vi "Get NIPKG Attributes from VIPM Package File.vi"(6 "Category":string(combo)="Add-Ons", 8 "error in (no error)":errorcluster, 9 "LabVIEW version":string="18.0", 11 "Source VIPM package (.vip)":path) -> (0 "error out":errorcluster, 1 "LabVIEW version out":string="18.0", 2 "package attributes":T1={"Package Name"="", "Display name"="", "Version"="", "Display version"="", "Synopsis"="", "Description"="", "Maintainer"="", "Maintainer email address"="", "Category"="", "Homepage"="", "Release notes"="", "Depends"=[], "Recommends"=[], "Suggests"=[], "Conflicts"=[], "Provides"=[], "Replaces"=[], "Supplements"=[], "Enhances"=[], "Product"=FALSE, "User visible"=FALSE, "Installed size (KB)"=0, "Package filesize (bytes)"=0, "Architecture"="", "Agent"="file", "MD5Checksum"=""}, 3 "VIPM Package Installed Filepaths":path[](array[path]), 4 "VIPM dependencies":string[](array[string]))   [LabVIEW 2014, in "vipm-to-nipm-package-converter.lvlib"]
doc: "From the specified VIPM package (.vip), convert the package attributes into the NIPM package attribute format and return the corresponding NIPM package attributes and return the installed filepaths of the VIPM package.\n\nINPUT(S):\n<b>LabVIEW version</b>: Specifies the LabVIEW version for the NIPM package to support (\"14.0\", \"14.0 (64-bit)\", \"18.0\", \"18.0 (64-bit)\", etc)"
uses:
  vipm-to-nipm-package-converter.lvlib
  <vilib>/National Instruments/NIPM API (Beta)/_support/package attributes.ctl
  <vilib>/Utility/config.llb/Read Key (String).vi
  <vilib>/Utility/config.llb/NI_LVConfig.lvlib
  <vilib>/National Instruments/NIPM API (Beta)/NIPM_API.lvlib
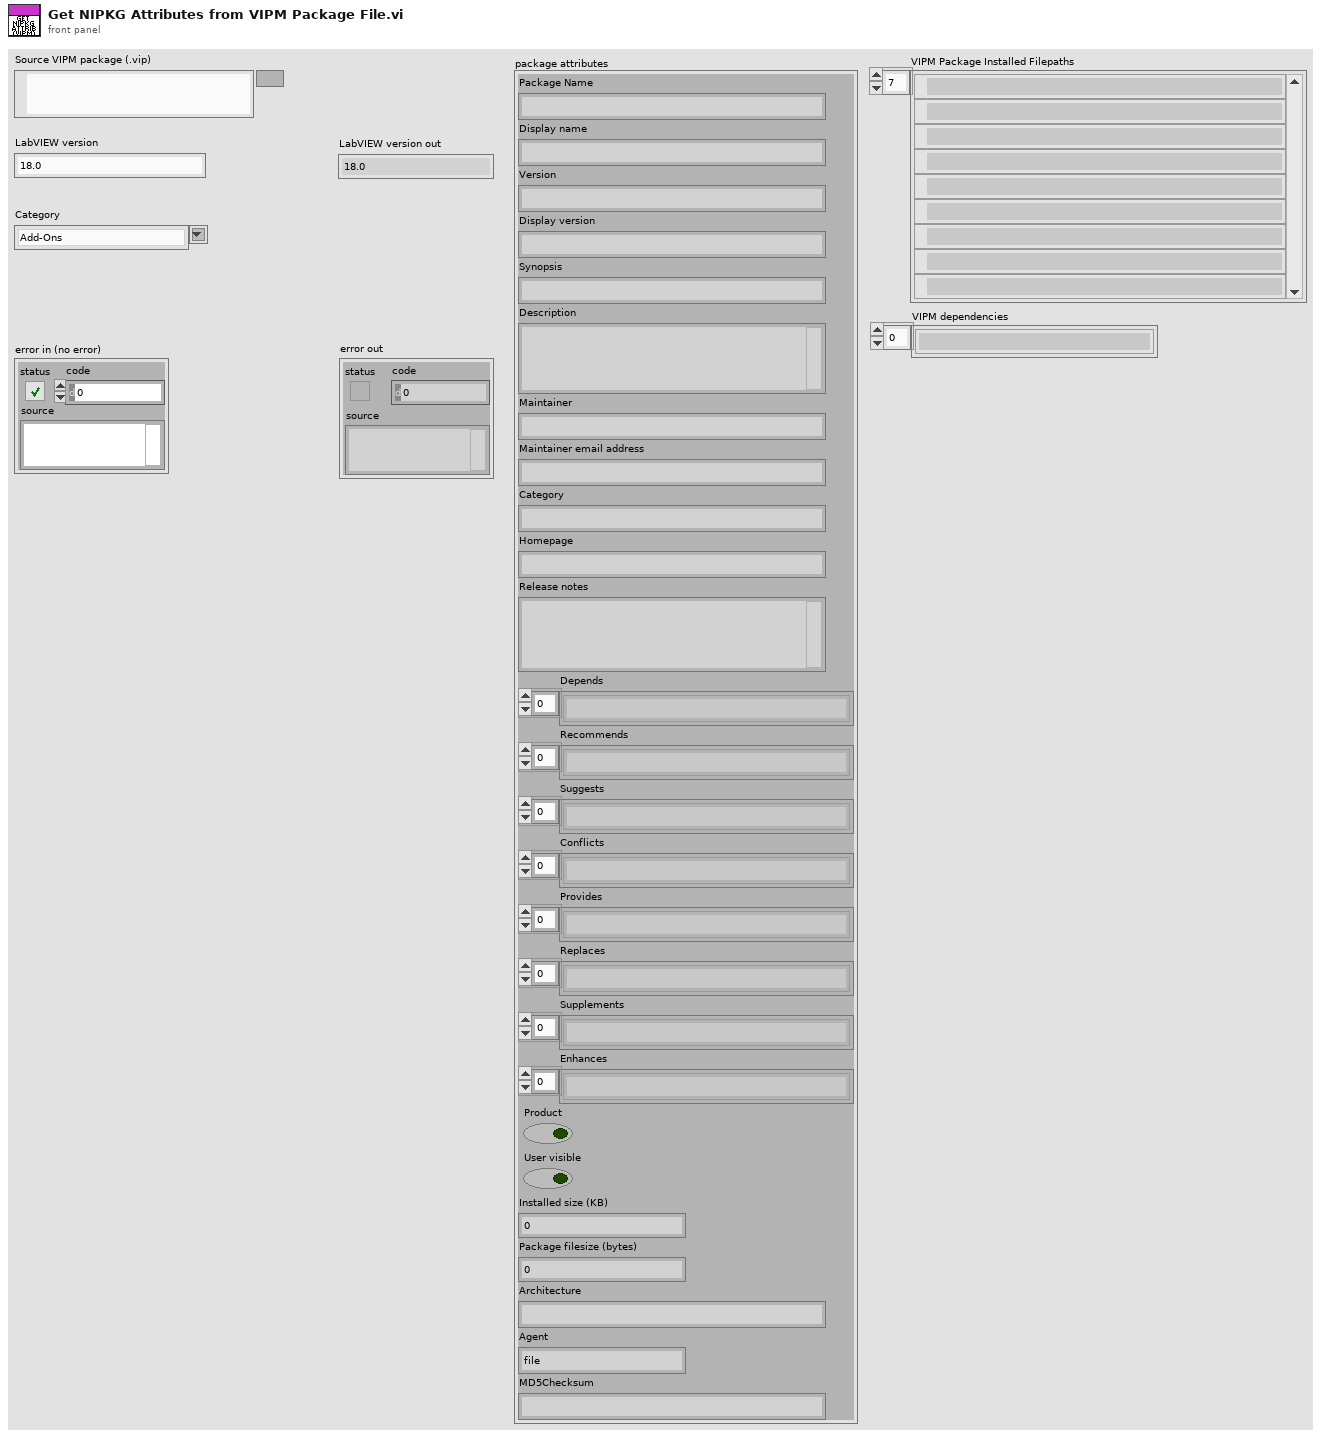
[diagram p1: front panel]
types:
  T1 = typedef "NIPM_API.lvlib/package attributes.ctl" = cluster{"Package Name":string, "Display name":string, "Version":string, "Display version":string, "Synopsis":string, "Description":string, "Maintainer":string, "Maintainer email address":string, "Category":string, "Homepage":string, "Release notes":string, "Depends":string[], "Recommends":string[], "Suggests":string[], "Conflicts":string[], "Provides":string[], "Replaces":string[], "Supplements":string[], "Enhances":string[], "Product":bool, "User visible":bool, "Installed size (KB)":u64, "Package filesize (bytes)":u64, "Architecture":string, "Agent":string, "MD5Checksum":string}
  T2 = typedef "NI_LVConfig.lvlib/Config Data RefNum.ctl" = refnum<k1>
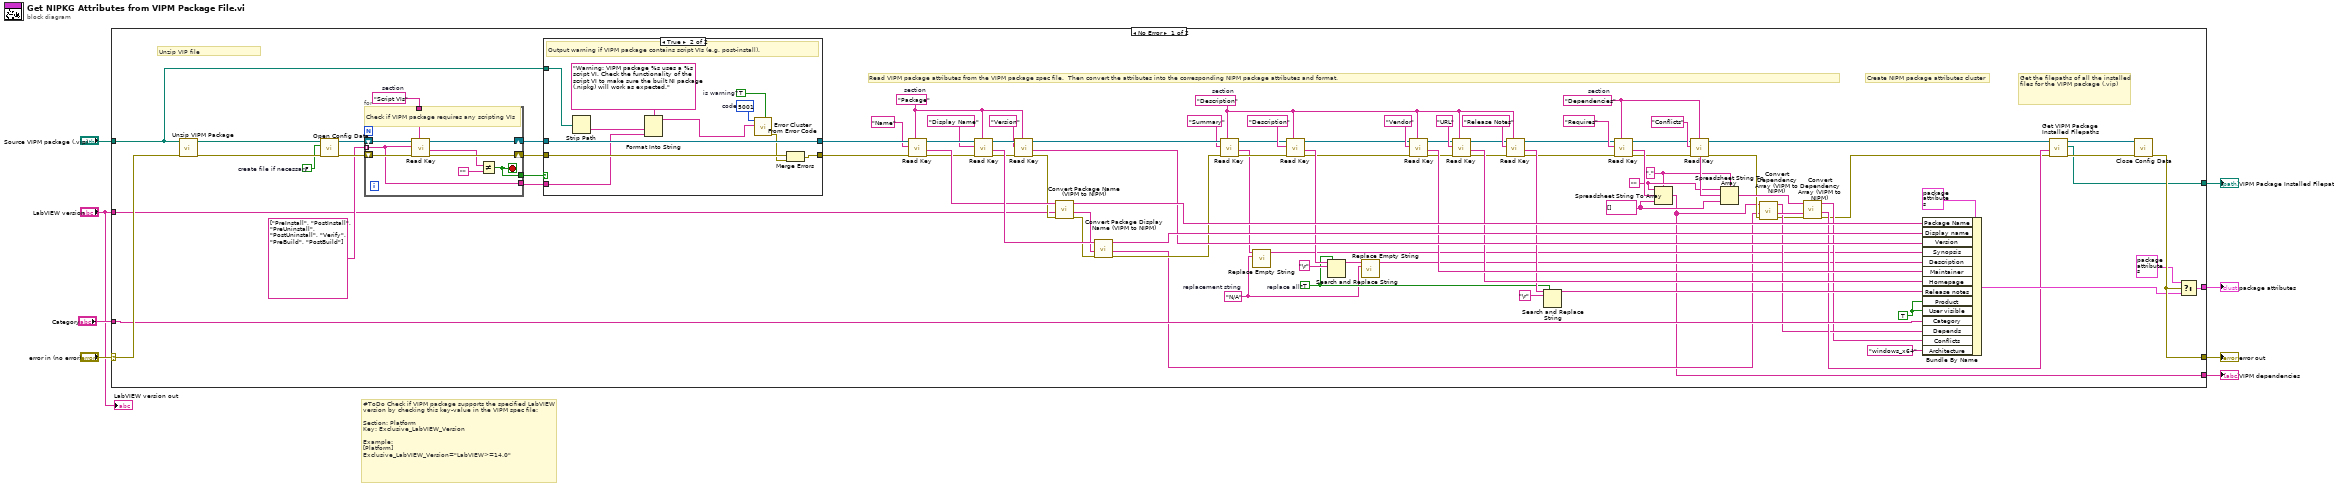
[diagram p0: block diagram]
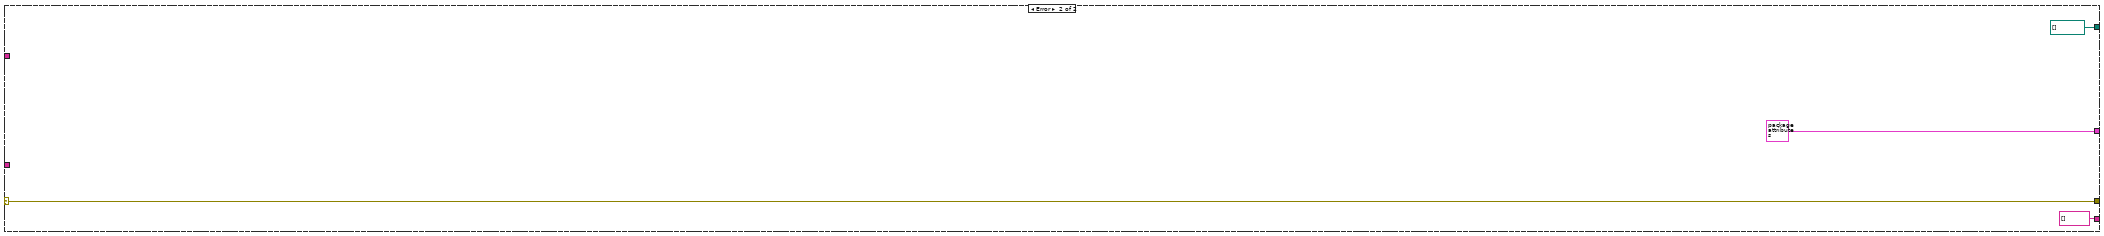
[diagram p3: hidden frame]
diagram:
  # "#ToDo Check if VIPM package supports the specified LabVIEW version by checking this key-value in the VIPM spec file:\n\nSection: Platform\nKey: Exclusive_LabVIEW_Version\n\nExample:\n[Platform]\nExclusive_LabVIEW_Version=\"LabVIEW>=14.0\""
  n1 = case shown="No Error" "error in (no error)" {
    selector: "error in (no error)" -> [w100 w129]
    tunnel: [w93 T1 {"Package Name"="", "Display name"="", "Version"="", "Display version"="", "Synopsis"="", "Description"="", "Maintainer"="", "Maintainer email address"="", "Category"="", "Homepage"="", "Release notes"="", "Depends"=[], "Recommends"=[], "Suggests"=[], "Conflicts"=[], "Provides"=[], "Replaces"=[], "Supplements"=[], "Enhances"=[], "Product"=FALSE, "User visible"=FALSE, "Installed size (KB)"=0, "Package filesize (bytes)"=0, "Architecture"="", "Agent"="file", "MD5Checksum"=""} ("package attributes")] -> w8
    tunnel: "LabVIEW version" -> [w12 _]
    tunnel: "Source VIPM package (.vip)" -> [w81 _]
    tunnel: [w96 w129] -> w6
    tunnel: "Category" -> [w99 _]
    tunnel: [w88 path[] [] ("Installed Filepaths")] -> w2
    tunnel: [w9 string[] []] -> w1
    frame No Error {
      w15 = "N/A"  # replacement string
      w34 = string[] []
      w35 = ""
      w28 = "," ("delimiter (Tab)")
      w39 = "Dependencies"  # section
      w43 = TRUE  # replace all?
      w52 = TRUE ("Product")
      w61 = "Description"  # section
      w72 = "Package"  # section
      w90 = "Script VIs"  # section
      w101 = FALSE  # create file if necessary
      # "Get the filepaths of all the installed files for the VIPM package (.vip)"
      # "Create NIPM package attributes cluster"
      # "Read VIPM package attributes from the VIPM package spec file.  Then convert the attributes into the corresponding NIPM package attributes and format."
      # "Unzip VIP file"
      n2 = call "Unzip VIPM Package.vi"("error in (no error)"=w100, "Source VIPM package (.vip)"=w81) -> ("error out"=w103:errorcluster, "VIPM package spec filepath"=w102:path)  [unwired: 8 in]
      n3 = call <vilib>:"Open Config Data.vi"("error in (no error)"=w103, "create file if necessary (T)"=w101, "configuration file path"=w102) -> ("error out"=w91:errorcluster, "refnum"=w92:T2)  [unwired: 6 in, 1 out]
      n4 = for {
        tunnel: w90 -> [w121]
        shift-right: [w123] -> w86
        shift-left: w92 -> [w125]
        shift-right: [w122] -> w84
        shift-left: w91 -> [w124]
        tunnel: string[] ["PreInstall", "PostInstall", "PreUninstall", "PostUninstall", "Verify", "PreBuild", "PostBuild"] -> [w118] mode=indexing
        tunnel: [w119] -> w87
        tunnel: [w118] -> w82
        stop <- w119 stop-if-true
        # "Check if VIPM package requires any scripting VIs"
        n5 = call-poly <vilib>:"Read Key.vi"("section"=w121, "error in (no error)"=w124, "key"=w118, "refnum"=w125) -> ("error out"=w122:errorcluster, "value"=w117:string, "refnum out"=w123:T2)  [unwired: 4 in, 1 out]
        n6 = Not Equal?(x=w117, y="") -> (x != y?=w119:bool)
      }
      n7 = case shown="True" w87 {
        tunnel: w86 -> [w105 w116]
        tunnel: [w105 w116] -> w85
        tunnel: w84 -> [w104 w115]
        tunnel: [w104 w108] -> w83
        tunnel: w82 -> [_ w111]
        tunnel: w81 -> [_ w112]
        frame False {
          # "VIPM package does not contain any script VIs"
        }
        frame True {
          w106 = TRUE  # is warning?
          w110 = 5001  # code
          # "Output warning if VIPM package contains script VIs (e.g. post-install)."
          n8 = Strip Path(path=w112) -> (name=w114:string)  [unwired: 1 out]
          n9 = Format Into String(format string="Warning: VIPM package %s uses a %s script VI. Check the functionality of the script VI to make sure the built NI package (.nipkg) will work as expected.", w114, w111) -> (resulting string=w109:string)  [unwired: 2 in, 1 out]
          n10 = call <vilib>:"Error Cluster From Error Code.vi"("is warning? (False)"=w106, "error message (\"\")"=w109, "error code (0)"=w110) -> ("error out"=w107:errorcluster)  [unwired: 6 in]
          n11 = Merge Errors(w115, w107) -> (w108:errorcluster)
        }
      }
      n12 = call-poly <vilib>:"Read Key.vi"("section"=w72, "error in (no error)"=w83, "key"="Name", "refnum"=w85) -> ("error out"=w42:errorcluster, "value"=w49:string, "refnum out"=w78:T2)  [unwired: 4 in, 1 out]
      n13 = call-poly <vilib>:"Read Key.vi"("section"=w72, "error in (no error)"=w42, "key"="Display Name", "refnum"=w78) -> ("error out"=w59:errorcluster, "value"=w75:string, "refnum out"=w73:T2)  [unwired: 4 in, 1 out]
      n14 = call-poly <vilib>:"Read Key.vi"("section"=w72, "error in (no error)"=w59, "key"="Version", "refnum"=w73) -> ("error out"=w41:errorcluster, "value"=w70:string, "refnum out"=w69:T2)  [unwired: 4 in, 1 out]
      n15 = call "Convert Package Name (VIPM to NIPM).vi"("error in (no error)"=w41, "LabVIEW version in"=w12, "VIPM Package Name"=w49) -> ("error out"=w51:errorcluster, "LabVIEW version out"=w11:string, "NIPM Package Name"=w76:string)  [unwired: 6 in]
      n16 = call "Convert Package Display Name (VIPM to NIPM).vi"("error in (no error)"=w51, "LabVIEW version in"=w11, "VIPM Package Display Name"=w75) -> ("error out"=w50:errorcluster, "LabVIEW version out"=w10:string, "NIPM Package Display Name"=w74:string)  [unwired: 6 in]
      n17 = call-poly <vilib>:"Read Key.vi"("section"=w61, "error in (no error)"=w50, "key"="Summary", "refnum"=w69) -> ("error out"=w58:errorcluster, "value"=w17:string, "refnum out"=w66:T2)  [unwired: 4 in, 1 out]
      n18 = call "Replace Empty String.vi"("replacement string"=w15, "string in"=w17) -> ("string out"=w16:string)  [unwired: 9 in]
      n19 = call-poly <vilib>:"Read Key.vi"("section"=w61, "error in (no error)"=w58, "key"="Description", "refnum"=w66) -> ("error out"=w18:errorcluster, "value"=w48:string, "refnum out"=w55:T2)  [unwired: 4 in, 1 out]
      n20 = Search and Replace String(replace all?=w43, input string=w48, search string="\r") -> (result string=w14:string)  [unwired: 5 in, 3 out]
      n21 = call "Replace Empty String.vi"("replacement string"=w15, "string in"=w14) -> ("string out"=w13:string)  [unwired: 9 in]
      n22 = call-poly <vilib>:"Read Key.vi"("section"=w61, "error in (no error)"=w18, "key"="Vendor", "refnum"=w55) -> ("error out"=w57:errorcluster, "value"=w64:string, "refnum out"=w54:T2)  [unwired: 4 in, 1 out]
      n23 = call-poly <vilib>:"Read Key.vi"("section"=w61, "error in (no error)"=w57, "key"="URL", "refnum"=w54) -> ("error out"=w56:errorcluster, "value"=w60:string, "refnum out"=w53:T2)  [unwired: 4 in, 1 out]
      n24 = call-poly <vilib>:"Read Key.vi"("section"=w61, "error in (no error)"=w56, "key"="Release Notes", "refnum"=w53) -> ("error out"=w30:errorcluster, "value"=w45:string, "refnum out"=w33:T2)  [unwired: 4 in, 1 out]
      n25 = Search and Replace String(replace all?=w43, input string=w45, search string="\r") -> (result string=w44:string)  [unwired: 5 in, 3 out]
      n26 = call-poly <vilib>:"Read Key.vi"("section"=w39, "error in (no error)"=w30, "key"="Requires", "refnum"=w33) -> ("error out"=w29:errorcluster, "value"=w37:string, "refnum out"=w32:T2)  [unwired: 4 in, 1 out]
      n27 = Spreadsheet String To Array(delimiter (Tab)=w28, format string=w35, spreadsheet string=w37, array type (2D Dbl)=w34) -> (array=w9:string[])
      n28 = call-poly <vilib>:"Read Key.vi"("section"=w39, "error in (no error)"=w29, "key"="Conflicts", "refnum"=w32) -> ("error out"=w20:errorcluster, "value"=w36:string, "refnum out"=w31:T2)  [unwired: 4 in, 1 out]
      n29 = Spreadsheet String To Array(delimiter (Tab)=w28, format string=w35, spreadsheet string=w36, array type (2D Dbl)=w34) -> (array=w27:string[])
      n30 = call "Convert Dependency Array (VIPM to NIPM).vi"("error in (no error)"=w20, "LabVIEW version in"=w10, "VIPM dependency string array"=w9) -> ("error out"=w21:errorcluster, "LabVIEW version out"=w26:string, "NIPM dependency string array"=w24:string[])  [unwired: 6 in]
      n31 = call "Convert Dependency Array (VIPM to NIPM).vi"("error in (no error)"=w21, "LabVIEW version in"=w26, "VIPM dependency string array"=w27) -> ("error out"=w19:errorcluster, "LabVIEW version out"=w25:string, "NIPM dependency string array"=w22:string[])  [unwired: 6 in]
      n32 = Bundle By Name(cluster=T1 {"Package Name"="", "Display name"="", "Version"="", "Display version"="", "Synopsis"="", "Description"="", "Maintainer"="", "Maintainer email address"="", "Category"="", "Homepage"="", "Release notes"="", "Depends"=[], "Recommends"=[], "Suggests"=[], "Conflicts"=[], "Provides"=[], "Replaces"=[], "Supplements"=[], "Enhances"=[], "Product"=FALSE, "User visible"=FALSE, "Installed size (KB)"=0, "Package filesize (bytes)"=0, "Architecture"="", "Agent"="file", "MD5Checksum"=""} ("package attributes"), "Package Name"=w76, "Display name"=w74, "Version"=w70, "Synopsis"=w16, "Description"=w13, "Maintainer"=w64, "Homepage"=w60, "Release notes"=w44, "Product"=w52, "User visible"=w52, "Category"=w99, "Depends"=w24, "Conflicts"=w22, "Architecture"="windows_x64") -> (w94:T1)
      n33 = call "Get VIPM Package Installed Filepaths.vi"("error in (no error)"=w19, "LabVIEW version in"=w25, "spec INI refnum in"=w31) -> ("error out"=w98:errorcluster, "Installed Filepaths"=w88:path[], "spec INI refnum out"=w97:T2)  [unwired: 5 in, 1 out]
      n34 = call <vilib>:"Close Config Data.vi"("error in (no error)"=w98, "refnum"=w97) -> ("error out"=w96:errorcluster)  [unwired: 8 in, 1 out]
      n35 = Select(t=T1 {"Package Name"="", "Display name"="", "Version"="", "Display version"="", "Synopsis"="", "Description"="", "Maintainer"="", "Maintainer email address"="", "Category"="", "Homepage"="", "Release notes"="", "Depends"=[], "Recommends"=[], "Suggests"=[], "Conflicts"=[], "Provides"=[], "Replaces"=[], "Supplements"=[], "Enhances"=[], "Product"=FALSE, "User visible"=FALSE, "Installed size (KB)"=0, "Package filesize (bytes)"=0, "Architecture"="", "Agent"="file", "MD5Checksum"=""}, s=w96, f=w94) -> (s? t:f=w93:T1)
    }
    frame Error {
    }
  }
  "package attributes" <- w8
  "error out" <- w6
  "VIPM Package Installed Filepaths" <- w2
  "VIPM dependencies" <- w1
  "LabVIEW version out" <- "LabVIEW version"
